vi "shortcutMenuClicked.vi"(8 "error in (no error)":errorcluster, 10 "MenuRef":refnum<k9>, 11 "ExperimentRunner in":refnum<class "ExperimentRunner.lvclass">) -> (0 "error out":errorcluster, 3 "ExperimentRunner out":refnum<class "ExperimentRunner.lvclass">)   [LabVIEW 2009, in "Views.lvlib" / "ExperimentControl.lvlib" / "ExperimentRunner.lvclass"]
uses:
  ExperimentRunner.lvclass
  MatlabScripts/MatlabScripts.lvclass
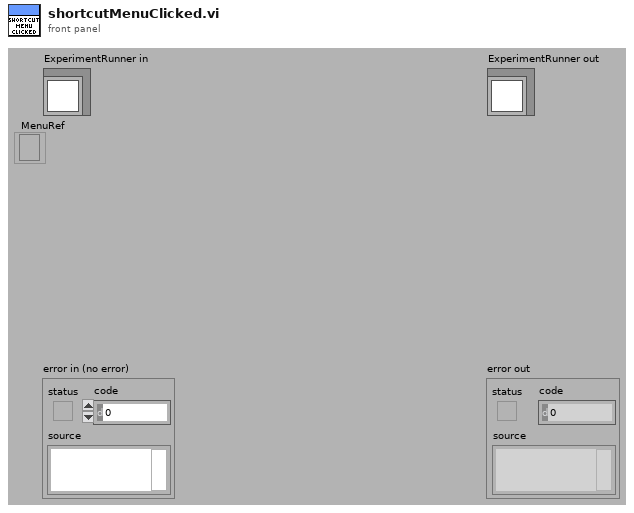
[diagram p1: front panel]
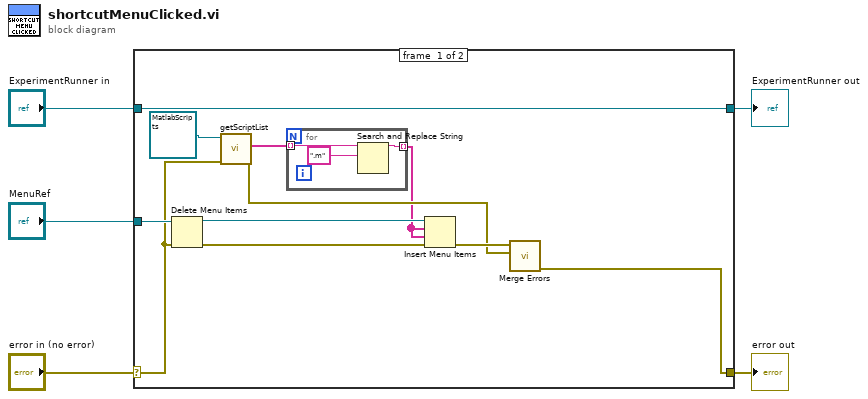
[diagram p0: block diagram]
diagram:
  n1 = case shown="No Error" "error in (no error)" {
    selector: "error in (no error)" -> [w13 w21]
    tunnel: [w8 w21] -> w4
    tunnel: [w16 w20] -> w2
    tunnel: "ExperimentRunner in" -> [w16 w20]
    tunnel: "MenuRef" -> [w15 _]
    frame #0 {
      n2 = Delete Menu Items(6:w13, 9:w15) -> (0:w11:errorcluster, 3:w12:refnum<k9>)  [unwired: 2 in]
      n3 = call "getScriptList.vi"("error in (no error)"=w13, "MatlabScripts in"=refnum<class "MatlabScripts.lvclass"> refnum ("Views.lvlib:ExperimentControl.lvlib:MatlabScripts.lvclass")) -> ("error out"=w9:errorcluster, "scriptNames"=w7:string[])  [unwired: 7 in, 1 out]
      n4 = for {
        tunnel: w7 -> [w19] mode=indexing
        tunnel: [w17] -> w6 mode=indexing
        n5 = Search and Replace String(input string=w19, search string=".m") -> (result string=w17:string)  [unwired: 6 in, 3 out]
      }
      n6 = Insert Menu Items(6:w11, 7:w6, 8:w6, 9:w12) -> (0:w10:errorcluster)  [unwired: 2 in, 2 out]
      n7 = call <vilib>:"Merge Errors.vi"("error in 2 (no error)"=w9, "error in 1 (no error)"=w10) -> ("error out"=w8:errorcluster)  [unwired: 5 in]
    }
    frame #1 {
    }
  }
  "error out" <- w4
  "ExperimentRunner out" <- w2
